vi "Pick a New Target.vi"(0 "Focus and Tracking":T4, 1 "System of Reference Interface":T5, 2 "Calibration":T6, 3 "Target":T3, 4 "Tip":T2, 5 "Error In":errorcluster, 6 "Refocus Step [um]":dbl=4.0, 7 "Frames per plane":i32=3, 8 "Z direction":i8(ring)=-1 items=["Positive"=1, "Negative"=-1], 10 "Minimal Clearance [um]":dbl=4.0, 11 "Active":refnum<vi>, 12 "Max Distance [um]":dbl=100.0, 13 "Abort":refnum<vi>) -> (14 "Target Coordinates":T1, 15 "Done":bool, 16 "Fail":bool, 17 "Scope Error":bool, 19 "Error Out":errorcluster)   [LabVIEW 2012, in "Targeting Unit.lvlib"]
uses:
  Targeting Unit.lvlib
  <vilib>/Analysis/Matrix/Datatypes/RealMatrix.ctl
  <vilib>/Analysis/Matrix/NI_Matrix.lvlib
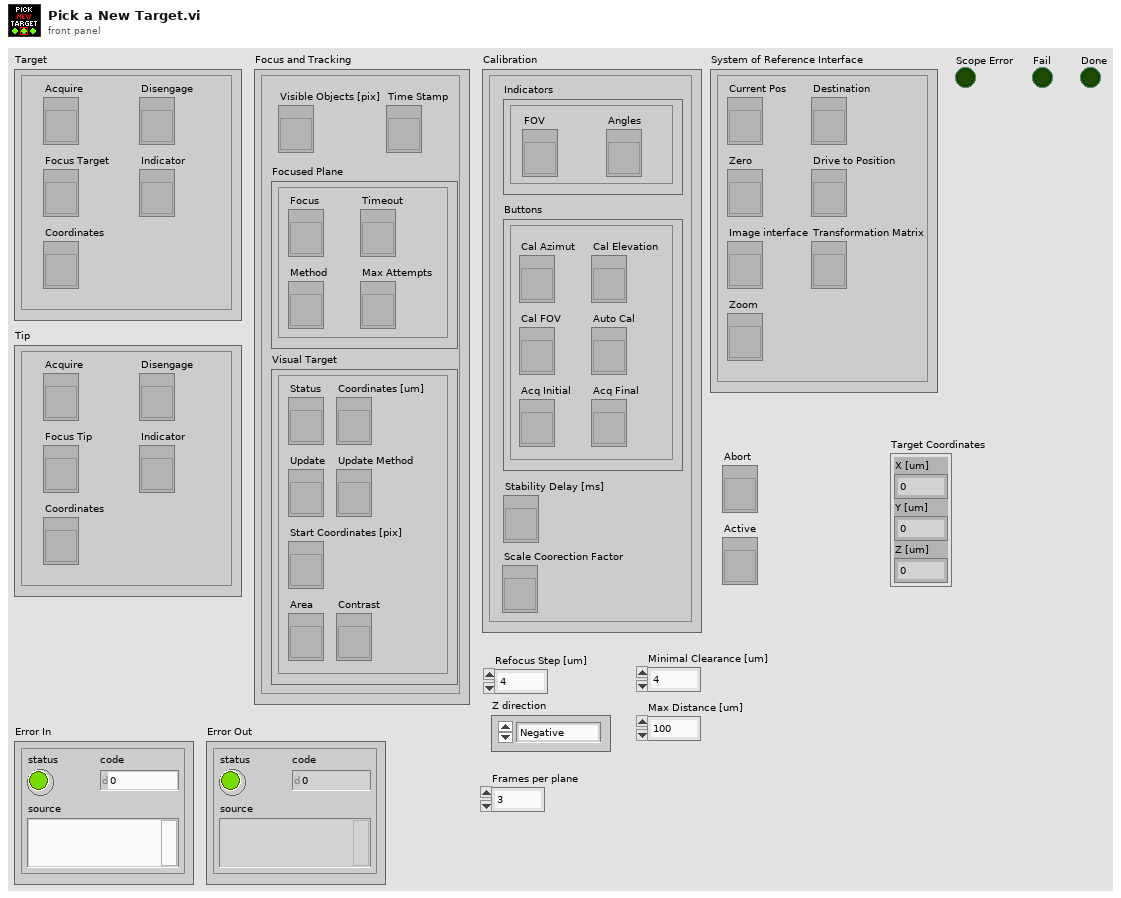
[diagram p1: front panel]
types:
  T1 = cluster{"X [um]":dbl, "Y [um]":dbl, "Z [um]":dbl}
  T2 = cluster{"Coordinates":refnum<vi>, "Acquire":refnum<vi>, "Disengage":refnum<vi>, "Indicator":refnum<vi>, "Focus Tip":refnum<vi>}
  T3 = cluster{"Coordinates":refnum<vi>, "Acquire":refnum<vi>, "Disengage":refnum<vi>, "Indicator":refnum<vi>, "Focus Target":refnum<vi>}
  T4 = cluster{"Focused Plane":cluster{"Focus":refnum<vi>, "Timeout":refnum<vi>, "Max Attempts":refnum<vi>, "Method":refnum<vi>}, "Time Stamp":refnum<vi>, "Visual Target":cluster{"Coordinates [um]":refnum<vi>, "Status":refnum<vi>, "Update":refnum<vi>, "Update Method":refnum<vi>, "Start Coordinates [pix]":refnum<vi>, "Area":refnum<vi>, "Contrast":refnum<vi>}, "Visible Objects [pix]":refnum<vi>}
  T5 = cluster{"Current Pos":refnum<vi>, "Image interface":refnum<vi>, "Transformation Matrix":refnum<vi>, "Zero":refnum<vi>, "Destination":refnum<vi>, "Drive to Position":refnum<vi>, "Zoom":refnum<vi>}
  T6 = cluster{"Indicators":cluster{"FOV":refnum<vi>, "Angles":refnum<vi>}, "Buttons":cluster{"Cal FOV":refnum<vi>, "Cal Azimut":refnum<vi>, "Cal Elevation":refnum<vi>, "Auto Cal":refnum<vi>, "Acq Initial":refnum<vi>, "Acq Final":refnum<vi>}, "Stability Delay [ms]":refnum<vi>, "Scale Coorection Factor":refnum<vi>}
  T7 = cluster{"X [um]":dbl, "Y [um]":dbl, "Z [um]":dbl}[][]
  T8 = cluster{"Area":dbl, "Centre of Mass":cluster{"X":dbl, "Y":dbl}, "Global Rectangle":cluster{"Left":dbl, "Top":dbl, "Right":dbl, "Bottom":dbl}, "Contrast":dbl}[][]
  T9 = cluster{"X [um]":dbl, "Y [um]":dbl, "Z [um]":dbl}[]
  T10 = cluster{"Area":dbl, "Centre of Mass":cluster{"X":dbl, "Y":dbl}, "Global Rectangle":cluster{"Left":dbl, "Top":dbl, "Right":dbl, "Bottom":dbl}, "Contrast":dbl}[]
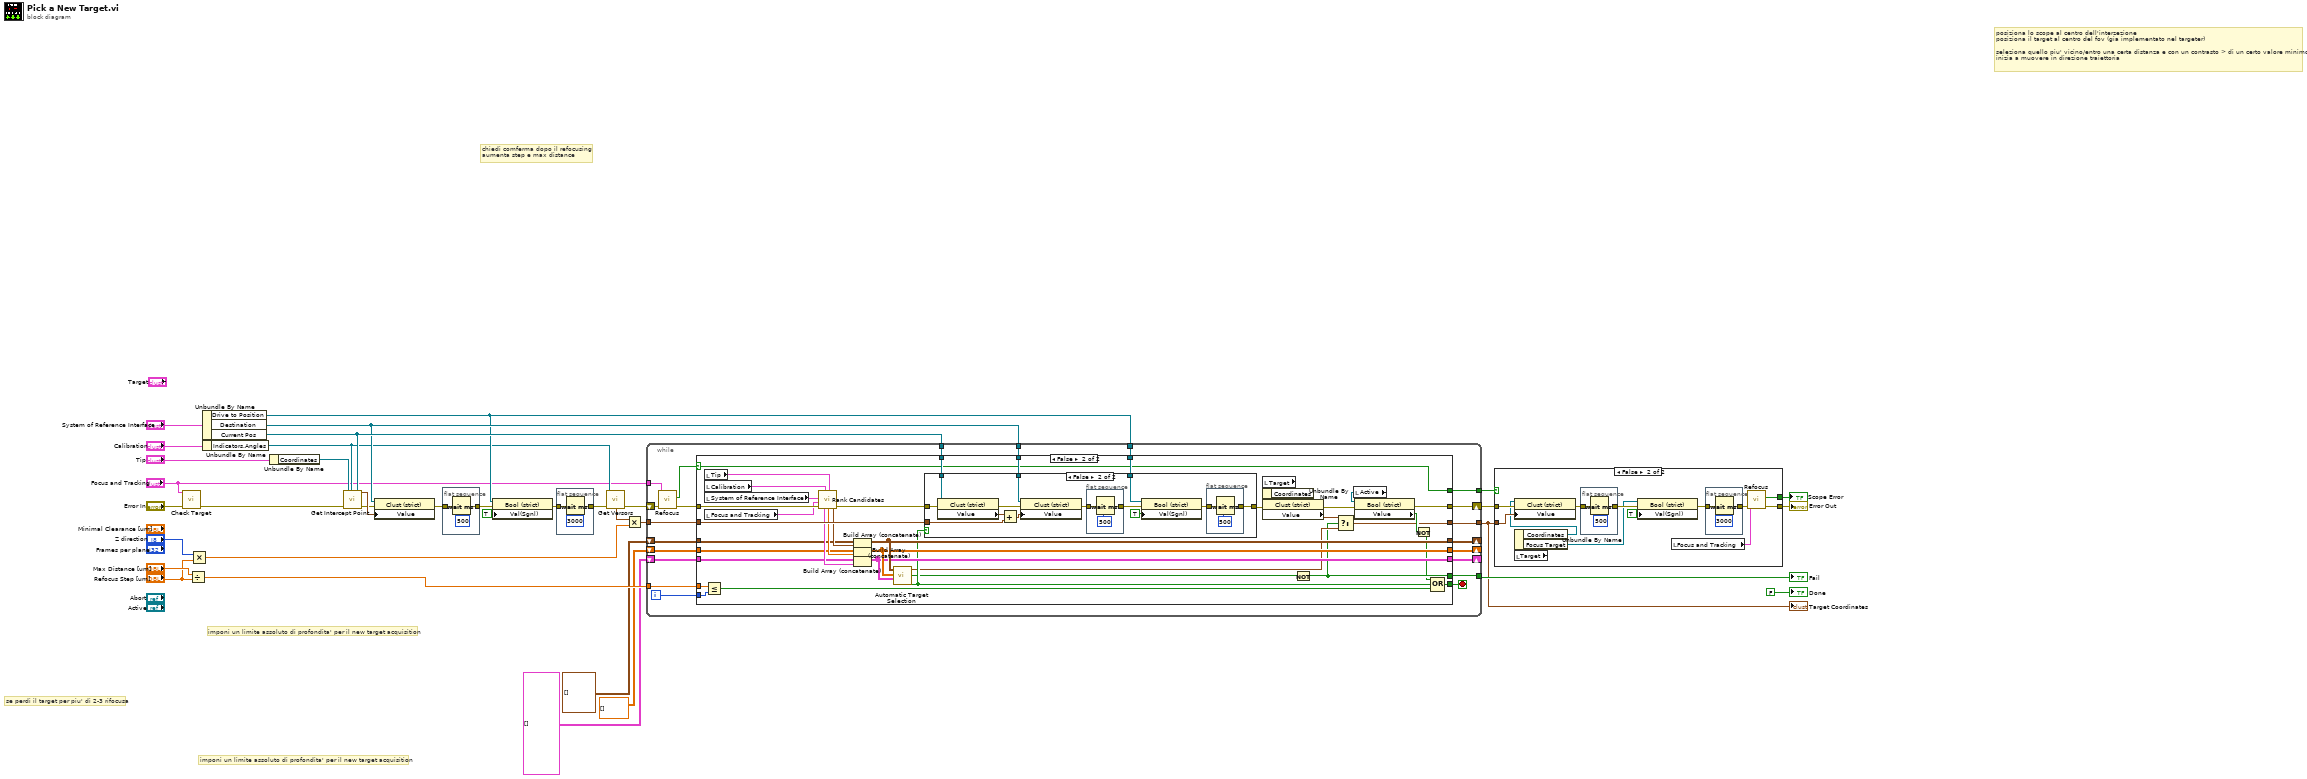
[diagram p0: block diagram]
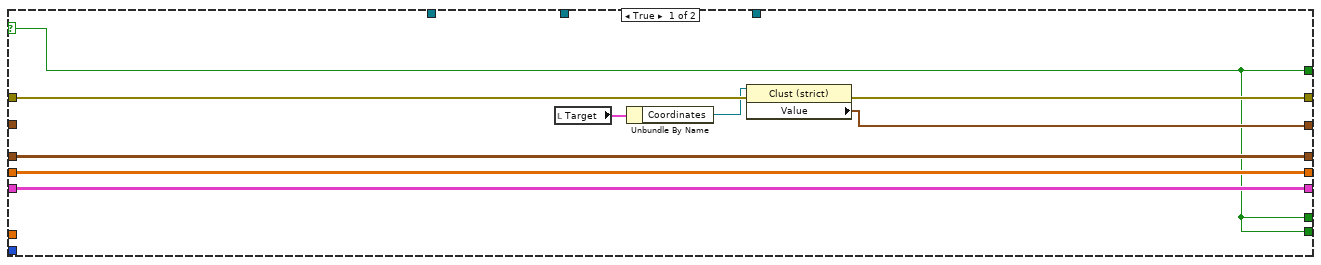
[diagram p3: hidden frame]
diagram:
  # "imponi un limite assoluto di profondita' per il new target acquisition"
  # "se perdi il target per piu' di 2-3 rifocusa"
  # "imponi un limite assoluto di profondita' per il new target acquisition"
  # "posiziona lo scope al centro dell'interzezione\nposiziona il target al centro del fov (gia implementato nel targeter)\n\nseleziona quello piu' vicino/entro una certa distanza e con un contrasto > di un certo valore minimo\ninizia a muovere in direzione traiettoria"
  # "chiedi comferma dopo il refocusing\naumenta step e max distance"
  n1 = call "Check Target.vi"("Error In"="Error In", "Focus and Tracking"="Focus and Tracking") -> ("Error out"=w2:errorcluster)  [unwired: 4 in, 5 out]
  n2 = Divide(x="Max Distance [um]", y="Refocus Step [um]") -> (x/y=w35:dbl)
  n3 = Multiply(x="Z direction", y="Refocus Step [um]") -> (x*y=w32:dbl)
  n4 = Unbundle By Name("System of Reference Interface") -> ("Drive to Position"=w7:refnum<vi>, "Destination"=w8:refnum<vi>, "Current Pos"=w12:refnum<vi>)
  n5 = Unbundle By Name("Calibration") -> ("Indicators.Angles"=w4:refnum<vi>)
  n6 = Unbundle By Name("Tip") -> ("Coordinates"=w3:refnum<vi>)
  n7 = call "Get Intercept Point.vi"("error in (no error)"=w2, "Current  System of Reference Position"=w12, "Tip Position"=w3, "Angles"=w4) -> ("error out"=w5:errorcluster, "Intercept Point"=w13:T1)  [unwired: 6 in]
  n8 = property class="Clust (strict)"(reference=w8, error in=w5, "Value"=w13) -> (error out=w18:errorcluster)  [unwired: 1 out]
  n9 = flat-sequence {
    tunnel: [w38] -> w17
    tunnel: w18 -> [w38]
    frame #0 {
      n10 = Wait (ms)(milliseconds to wait=u32 500) -> ()  [unwired: 1 out]
    }
  }
  n11 = property class="Bool (strict)"(reference=w7, error in=w17, "Val(Sgnl)"=TRUE ("Value")) -> (error out=w15:errorcluster)  [unwired: 1 out]
  n12 = flat-sequence {
    tunnel: [w40] -> w6
    tunnel: w15 -> [w40]
    frame #0 {
      n13 = Wait (ms)(milliseconds to wait=u32 3000) -> ()  [unwired: 1 out]
    }
  }
  n14 = call "Get Versors.vi"("error in (no error)"=w6, "Angles"=w4) -> ("error out"=w11:errorcluster, "Versor"=w14:cluster{"X":dbl, "Y":dbl, "Z":dbl})  [unwired: 8 in]
  n15 = Multiply(x=w14, y=w32) -> (x*y=w16:cluster{"X":dbl, "Y":dbl, "Z":dbl})
  n16 = while {
    tunnel: w16 -> [w58]
    tunnel: w8 -> [w61]
    tunnel: w7 -> [w60]
    tunnel: w12 -> [w59]
    shift-right: [w46] -> w10
    shift-left: w11 -> [w56]
    tunnel: "Focus and Tracking" -> [w42]
    tunnel: w35 -> [w49]
    shift-right: [w50] -> _
    shift-left: T8 [] -> [w55]
    shift-right: [w51] -> _
    shift-left: dbl[][] [] -> [w54]
    shift-right: [w52] -> _
    shift-left: T7 [] -> [w53]
    tunnel: [w47] -> w27
    tunnel: [w43] -> w9
    tunnel: [w41] -> w28
    i -> [w48]
    stop <- w45 stop-if-true
    n17 = call "Refocus.vi"("Error In"=w56, "Focus and Tracking"=w42) -> ("Error Out"=w57:errorcluster, "Error"=w44:bool)  [unwired: 8 in]
    n18 = case shown="False" w44 {
      selector: w44 -> [w64 w79]
      tunnel: w61 -> [_ w108]
      tunnel: w60 -> [_ w107]
      tunnel: w59 -> [_ w106]
      tunnel: w58 -> [_ w105]
      tunnel: w57 -> [w67 w104]
      tunnel: w55 -> [w70 w101]
      tunnel: w54 -> [w69 w99]
      tunnel: w53 -> [w68 w97]
      tunnel: [w68 w96] -> w52
      tunnel: [w69 w95] -> w51
      tunnel: [w70 w94] -> w50
      tunnel: w49 -> [_ w93]
      tunnel: w48 -> [_ w92]
      tunnel: [w65 w82] -> w47
      tunnel: [w66 w91] -> w46
      tunnel: [w64 w90] -> w45
      tunnel: [w64 w79] -> w43
      tunnel: [w64 w72] -> w41
      frame True {
        n19 = local read "Target"() -> (w63:T3)
        n20 = Unbundle By Name(w63) -> ("Coordinates"=w62:refnum<vi>)
        n21 = property class="Clust (strict)"(reference=w62, error in=w67) -> (error out=w66:errorcluster, "Value"=w65:T1)  [unwired: 1 out]
      }
      frame False {
        n22 = local read "Tip"() -> (w75:T2)
        n23 = local read "Calibration"() -> (w76:T6)
        n24 = local read "System of Reference Interface"() -> (w77:T5)
        n25 = local read "Focus and Tracking"() -> (w78:T4)
        n26 = Less Or Equal?(x=w93, y=w92) -> (x <= y?=w89:bool)
        n27 = call "Rank Candidates.vi"("Focus and Tracking"=w78, "System of Reference Interface"=w77, "Tip"=w75, "Calibration"=w76, "error in (no error)"=w104) -> ("Coords [um]"=w98:T9, "Scores"=w100:dbl[], "Visible Objects [pix]"=w102:T10, "error out"=w103:errorcluster)  [unwired: 7 in]
        n28 = Build Array (concatenate)(w97, w98) -> (w96:T7)
        n29 = Build Array (concatenate)(w99, w100) -> (w95:dbl[][])
        n30 = Build Array (concatenate)(w101, w102) -> (w94:T8)
        n31 = call "Automatic Target Selection.vi"("Visible Objects [pix]"=w94, "Scores"=w95, "Coords [um]"=w96) -> ("Stop"=w87:bool, "Target OK"=w86:bool, "Target Coordinates"=w81:T1)  [unwired: 6 in]
        n32 = case shown="False" w87 {
          tunnel: w108 -> [_ w119]
          tunnel: w107 -> [_ w115]
          tunnel: w106 -> [_ w114]
          tunnel: w105 -> [_ w112]
          tunnel: w103 -> [w109 w111]
          tunnel: [w109 w110] -> w84
          frame True {
          }
          frame False {
            n33 = property class="Clust (strict)"(reference=w114, error in=w111) -> (error out=w122:errorcluster, "Value"=w121:T1)  [unwired: 1 out]
            n34 = Add(x=w121, y=w112) -> (x+y=w120:cluster{dbl, dbl, dbl})
            n35 = property class="Clust (strict)"(reference=w119, error in=w122, "Value"=w120) -> (error out=w118:errorcluster)  [unwired: 1 out]
            n36 = flat-sequence {
              tunnel: [w126] -> w116
              tunnel: w118 -> [w126]
              frame #0 {
                n37 = Wait (ms)(milliseconds to wait=u32 500) -> ()  [unwired: 1 out]
              }
            }
            n38 = property class="Bool (strict)"(reference=w115, error in=w116, "Val(Sgnl)"=TRUE ("Value")) -> (error out=w113:errorcluster)  [unwired: 1 out]
            n39 = flat-sequence {
              tunnel: [w124] -> w110
              tunnel: w113 -> [w124]
              frame #0 {
                n40 = Wait (ms)(milliseconds to wait=u32 500) -> ()  [unwired: 1 out]
              }
            }
          }
        }
        n41 = local read "Target"() -> (w74:T3)
        n42 = Unbundle By Name(w74) -> ("Coordinates"=w73:refnum<vi>)
        n43 = property class="Clust (strict)"(reference=w73, error in=w84) -> (error out=w83:errorcluster, "Value"=w80:T1)  [unwired: 1 out]
        n44 = Not(x=w86) -> (.not. x?=w72:bool)
        n45 = Select(t=w80, s=w72, f=w81) -> (s? t:f=w82:T1)
        n46 = local read "Active"() -> (w85:refnum<vi>)
        n47 = property class="Bool (strict)"(reference=w85, error in=w83) -> (error out=w91:errorcluster, "Value"=w88:bool)  [unwired: 1 out]
        n48 = Not(x=w88) -> (.not. x?=w71:bool)
        n49 = Compound Arithmetic op=OR(w71, w87, w89) -> (w90:bool)
      }
    }
  }
  "Fail" <- w28
  "Target Coordinates" <- w27
  n50 = case shown="False" w9 {
    selector: w9 -> [w127 _]
    tunnel: w10 -> [w128 w141]
    tunnel: [w128 w129] -> w20
    tunnel: w27 -> [_ w132]
    tunnel: [w127 w130] -> w21
    frame True {
    }
    frame False {
      n51 = local read "Target"() -> (w140:T3)
      n52 = Unbundle By Name(w140) -> ("Coordinates"=w131:refnum<vi>, "Focus Target"=w134:refnum<vi>)
      n53 = property class="Clust (strict)"(reference=w131, error in=w141, "Value"=w132) -> (error out=w137:errorcluster)  [unwired: 1 out]
      n54 = flat-sequence {
        tunnel: [w145] -> w138
        tunnel: w137 -> [w145]
        frame #0 {
          n55 = Wait (ms)(milliseconds to wait=u32 500) -> ()  [unwired: 1 out]
        }
      }
      n56 = property class="Bool (strict)"(reference=w134, error in=w138, "Val(Sgnl)"=TRUE ("Value")) -> (error out=w136:errorcluster)  [unwired: 1 out]
      n57 = local read "Focus and Tracking"() -> (w133:T4)
      n58 = flat-sequence {
        tunnel: [w143] -> w135
        tunnel: w136 -> [w143]
        frame #0 {
          n59 = Wait (ms)(milliseconds to wait=u32 3000) -> ()  [unwired: 1 out]
        }
      }
      n60 = call "Refocus.vi"("Error In"=w135, "Focus and Tracking"=w133) -> ("Error Out"=w129:errorcluster, "Error"=w130:bool)  [unwired: 8 in]
    }
  }
  "Error Out" <- w20
  "Scope Error" <- w21
  "Done" <- FALSE
